vi "FTW-SQLite-Construct.vi"(0 "Database URI":string, 2 "Database Type":T1, 5 "Access Mode":T2, 11 "error in":errorcluster) -> (4 "SQLite Connector":refnum<class "FTW-SQLite-Connector.lvclass">, 6 "SQLite Version":string, 15 "error out":errorcluster)   [LabVIEW 2013, in "FTW-SQLite-Connector.lvclass"]
uses:
  FTW-SQLite-Connector.lvclass
  FTW-SQLite-AccessMode.ctl
  FTW-SQLite-DatabaseType.ctl
  FTW-SQLite-Connector.lvclass/FTW-SQLite-Connector.ctl
  error/FTW-ERR-ThrowGenericError.vi
  error/FTW-ERR-ThrowError.vi
  error/FTW-ERR-NoErrorConstant.vi
  error/FTW-ERR-CallChain.vi
  string/FTW-STR-ReplaceWhitespace.vi
panel:
  # "Inputs"
  # "Outputs"
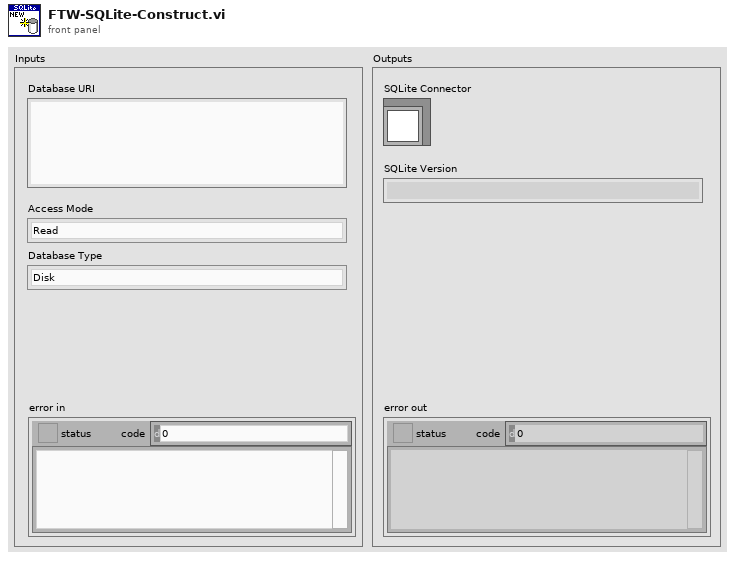
[diagram p1: front panel]
types:
  T1 = typedef "FTW-SQLite-Connector.lvclass/FTW-SQLite-DatabaseType.ctl" = enum16{"Disk", "Memory"}
  T2 = typedef "FTW-SQLite-Connector.lvclass/FTW-SQLite-AccessMode.ctl" = enum16{"Read", "Read/Write", "Read/Write/Create"}
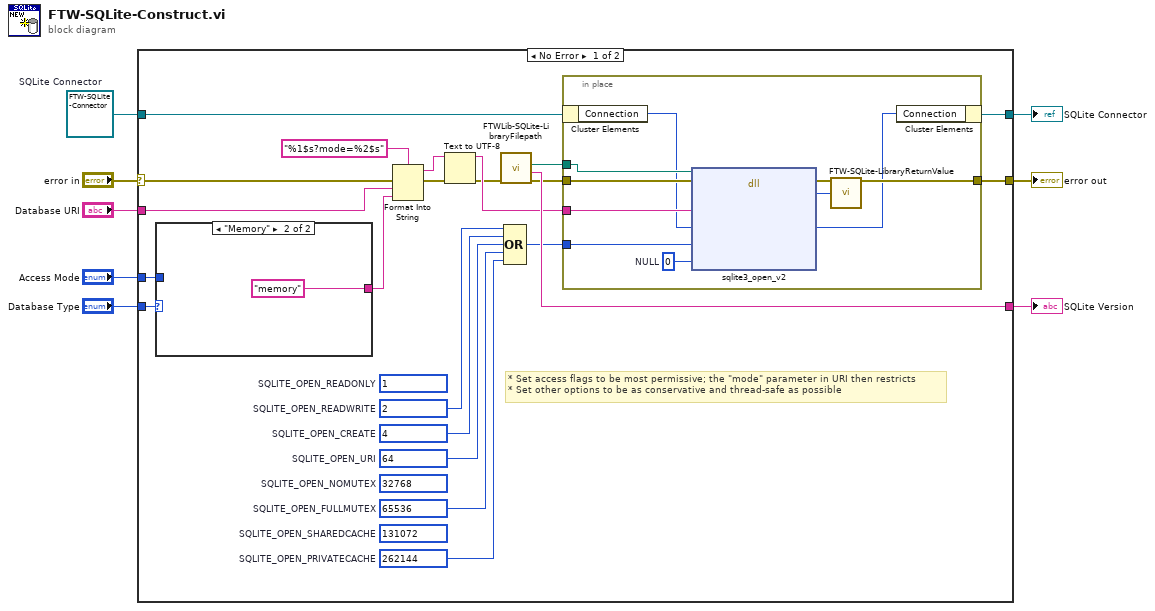
[diagram p0: block diagram]
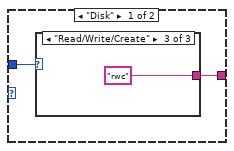
[diagram p2: hidden frame]
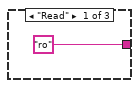
[diagram p3: hidden frame]
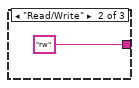
[diagram p4: hidden frame]
diagram:
  w7 = refnum<class "FTW-SQLite-Connector.lvclass"> refnum  # SQLite Connector
  n1 = case shown="No Error" "error in" {
    selector: "error in" -> [w15 w48]
    tunnel: [w29 w48] -> w8
    tunnel: [w27 w47] -> w6
    tunnel: w7 -> [w28 w47]
    tunnel: [w30 _] -> w4
    tunnel: "Database URI" -> [w22 _]
    tunnel: "Access Mode" -> [w24 _]
    tunnel: "Database Type" -> [w9 _]
    frame No Error {
      w10 = u32 262144  # SQLITE_OPEN_PRIVATECACHE
      (unwired) u32 131072  # SQLITE_OPEN_SHAREDCACHE
      w11 = u32 65536  # SQLITE_OPEN_FULLMUTEX
      (unwired) u32 32768  # SQLITE_OPEN_NOMUTEX
      w12 = u32 64  # SQLITE_OPEN_URI
      w13 = u32 4  # SQLITE_OPEN_CREATE
      w14 = u32 2  # SQLITE_OPEN_READWRITE
      (unwired) u32 1  # SQLITE_OPEN_READONLY
      # "* Set access flags to be most permissive; the \"mode\" parameter in URI then restricts\n* Set other options to be as conservative and thread-safe as possible"
      n2 = case shown="\"Memory\"" w9 {
        tunnel: w24 -> [w32 _]
        tunnel: [w31 "memory"] -> w21
        frame "Disk" {
          n3 = case shown="\"Read/Write/Create\"" w32 {
            tunnel: ["ro" "rw" "rwc"] -> w31
            frame "Read" {
            }
            frame "Read/Write" {
            }
            frame "Read/Write/Create" {
            }
          }
        }
        frame "Memory" {
        }
      }
      n4 = Format Into String(format string="%1$s?mode=%2$s", error in=w15, w22, w21) -> (resulting string=w19:string, error out=w16:errorcluster)  [unwired: 1 in]
      n5 = Text to UTF-8(8:w16, 11:w19) -> (0:w17:errorcluster, 3:w20:string)
      n6 = call "FTWLib-SQLite-LibraryFilepath.vi"("error in"=w17) -> ("error out"=w25:errorcluster, "SQLite Version"=w30:string, "SQLite Library Filepath"=w26:path)  [unwired: 8 in]
      n7 = Compound Arithmetic op=OR(w14, w13, w12, w11, w10) -> (w18:u32)
      n8 = in-place {
        in-place-border: w25 -> [w46]
        in-place-border: w26 -> [w45]
        in-place-border: [w39] -> w29
        in-place-border: w18 -> [w42]
        in-place-border: w20 -> [w41]
        w40 = 0  # NULL
        n9 = in-place-cluster #1(w28) -> ("Connection"=w37:u64)
        n10 = dll-call lib="?" fn="sqlite3_open_v2"(path in=w45, error in=w46, "Database URI"=w41, "Connection Handle"=w37, "Flags"=w42, "VFS Name"=w40) -> (error out=w44:errorcluster, "Return Value"=w43:i32, "Connection Handle"=w38:u64)  [unwired: 4 in, 1 out]
        n11 = call "FTW-SQLite-LibraryReturnValue.vi"("error in"=w44, "Return Value"=w43) -> ("error out"=w39:errorcluster)  [unwired: 13 in]
        n12 = in-place-cluster #1("Connection"=w38) -> (w27:refnum<class "FTW-SQLite-Connector.lvclass">)
      }
    }
    frame Error {
    }
  }
  "error out" <- w8
  "SQLite Connector" <- w6
  "SQLite Version" <- w4
